vi "Read control functions indices.vi"(11 "user tag bus module in":refnum<class "user tag bus module.lvclass">) -> (2 "control functions":T1[](array[typedef]) {"output range"."output low" format="%.2f"; "output range"."output high" format="%.2f"}, 3 "user tag bus module out":refnum<class "user tag bus module.lvclass">)   [LabVIEW 2013, in "user tag bus module.lvclass"]
doc: "This function is intended to enable easier testing. Tests can get the indices of data without having to perform the lookup a second time."
uses:
  user tag bus module.lvclass
  control module.ctl
  user tag bus module.lvclass/user tag bus module.ctl
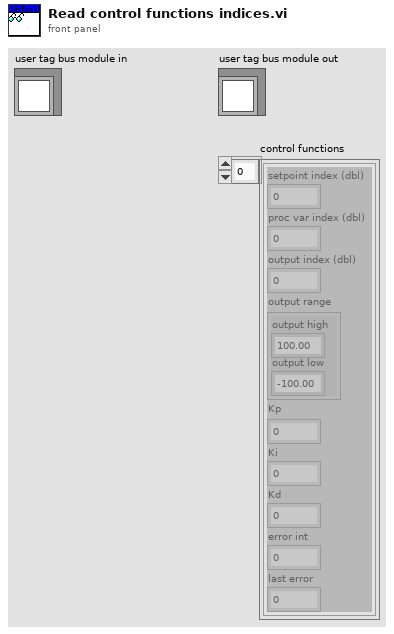
[diagram p1: front panel]
types:
  T1 = typedef "user tag bus module.lvclass/control module.ctl" = cluster{"setpoint index (dbl)":i32, "proc var index (dbl)":i32, "output index (dbl)":i32, "output range":cluster{"output high":dbl, "output low":dbl}, "Kp":dbl, "Ki":dbl, "Kd":dbl, "error int":dbl, "last error":dbl}
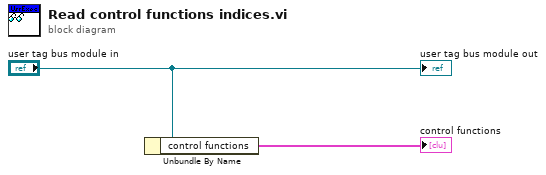
[diagram p0: block diagram]
diagram:
  n1 = Unbundle By Name("user tag bus module in") -> ("control functions"=→"control functions":T1[])
  "user tag bus module out" <- "user tag bus module in"
